vi "New Project.vi"(8 "error in (no error)":errorcluster, 10 "Path":path, 11 "Controller in":refnum<class "Controller.lvclass">) -> (0 "error out":errorcluster, 3 "Controller out":refnum<class "Controller.lvclass">)   [LabVIEW 2013, in "SET Project Editor.lvlib" / "Controller.lvclass"]
uses:
  Controller.lvclass
  Controller.lvclass/Controller.ctl
  Wizards/New Project Wizard/New Project Wizard.lvclass
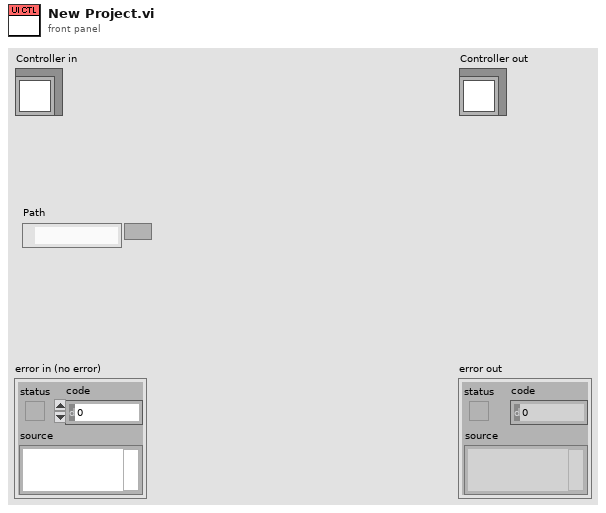
[diagram p1: front panel]
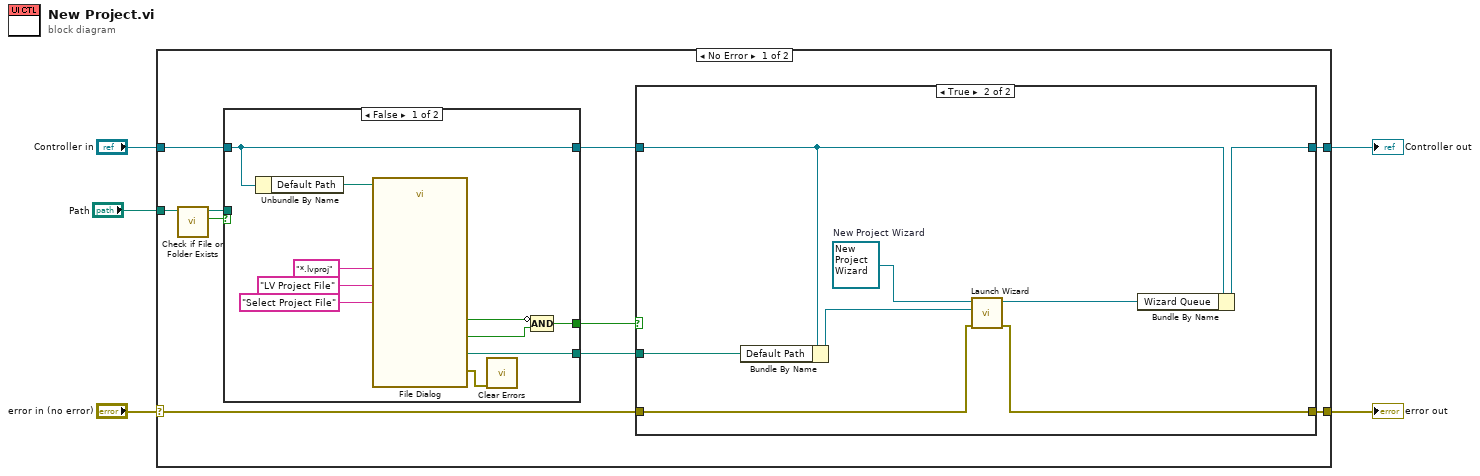
[diagram p0: block diagram]
diagram:
  n1 = case shown="No Error" "error in (no error)" {
    selector: "error in (no error)" -> [w11 w40]
    tunnel: [w15 w40] -> w4
    tunnel: [w14 w39] -> w2
    tunnel: "Controller in" -> [w7 w39]
    tunnel: "Path" -> [w10 _]
    frame No Error {
      n2 = call <vilib>:"Check if File or Folder Exists.vi"("path"=w10) -> ("file or folder exists?"=w8:bool, "dup path"=w9:path)  [unwired: 8 in, 1 out]
      n3 = case shown="False" w8 {
        selector: w8 -> [_ w26]
        tunnel: [w20 w27] -> w13
        tunnel: [w19 w26] -> w12
        tunnel: w9 -> [_ w27]
        tunnel: [w17 w28] -> w6
        tunnel: w7 -> [w17 w28]
        frame False {
          n4 = Unbundle By Name(w17) -> ("Default Path"=w16:path)
          n5 = call "File Dialog"("start path"=w16, "prompt"="Select Project File", "pattern (all files)"="*.lvproj", "pattern label"="LV Project File") -> ("selected path"=w20:path, "exists"=w22:bool, "cancelled"=w21:bool, "error out"=w18:errorcluster)  [unwired: 8 in]
          n6 = call <vilib>:"Clear Errors.vi"("error in (no error)"=w18) -> ()  [unwired: 6 in, 1 out]
          n7 = Compound Arithmetic op=AND(invert w21, w22) -> (w19:bool)
        }
        frame True {
        }
      }
      n8 = case shown="True" w12 {
        tunnel: [w29 w37] -> w15
        tunnel: w6 -> [w30 w36]
        tunnel: w13 -> [_ w34]
        tunnel: [w30 w38] -> w14
        tunnel: w11 -> [w29 w31]
        frame False {
        }
        frame True {
          w33 = refnum<class "New Project Wizard.lvclass"> refnum  # New Project Wizard
          n9 = Bundle By Name(cluster=w36, "Default Path"=w34) -> (w35:refnum<class "Controller.lvclass">)
          n10 = call-dynamic "Launch Wizard.vi"("error in (no error)"=w31, "Controller in"=w35, "New Project Wizard in"=w33) -> ("error out"=w37:errorcluster, "Caller-To-Actor Enqueuer"=w32:refnum<class "Message Enqueuer.lvclass">)  [unwired: 7 in]
          n11 = Bundle By Name(cluster=w36, "Wizard Queue"=w32) -> (w38:refnum<class "Controller.lvclass">)
        }
      }
    }
    frame Error {
    }
  }
  "error out" <- w4
  "Controller out" <- w2
